vi "Parse Session (Tx-Generic).vi"(8 "error in":errorcluster, 11 "node in":refnum<k20>) -> (0 "error out":errorcluster, 3 "tx_generic_setup":T1={"QueueSizeIn"=0, "Count"=12, "StartMode"=1} {"StartMode" items=["FDX_STOP", "FDX_START", "FDX_START_TRG", "FDX_START_TIME"]})   [LabVIEW 2020, in "AIM ARINC 664 Import.lvlib"]
uses:
  AIM ARINC 664 Import.lvlib
  _typedefs/tx_generic_setup.ctl
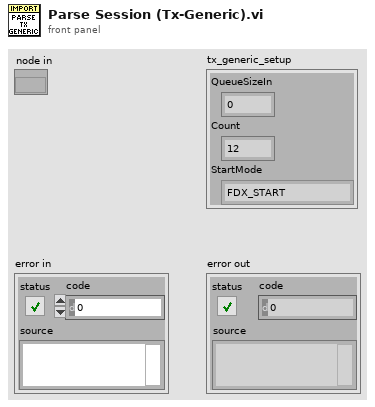
[diagram p1: front panel]
types:
  T1 = typedef "AIM ARINC 664 Import.lvlib/tx_generic_setup.ctl" = cluster{"QueueSizeIn":u32, "Count":i32, "StartMode":i32}
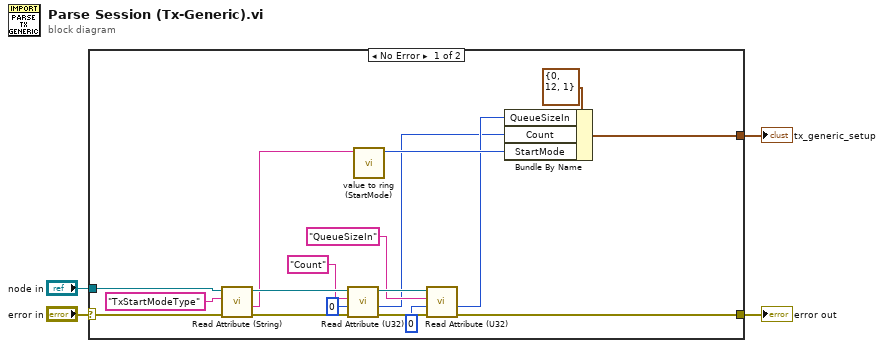
[diagram p0: block diagram]
diagram:
  n1 = case shown="No Error" "error in" {
    selector: "error in" -> [w16 w23]
    tunnel: "node in" -> [w19 _]
    tunnel: [w13 w23] -> w3
    tunnel: [w21 _] -> w1
    frame No Error {
      n2 = call "Read Attribute (String).vi"("error in"=w16, "Attribute Name"="TxStartModeType" ("Name"), "node in"=w19) -> ("error out"=w15:errorcluster, "value"=w7:string, "node out"=w18:refnum<k20>)  [unwired: 6 in]
      n3 = call "Read Attribute (U32).vi"("error in"=w15, "default"=u32 0, "Attribute Name"="Count" ("Tag Name"), "node in"=w18) -> ("error out"=w14:errorcluster, "value"=w8:u32, "node out"=w17:refnum<k20>)  [unwired: 5 in]
      n4 = call "value to ring (StartMode).vi"("value"=w7) -> ("StartMode"=w20:i32)  [unwired: 10 in]
      n5 = call "Read Attribute (U32).vi"("error in"=w14, "default"=u32 0, "Attribute Name"="QueueSizeIn" ("Tag Name"), "node in"=w17) -> ("error out"=w13:errorcluster, "value"=w9:u32)  [unwired: 5 in, 1 out]
      n6 = Bundle By Name(cluster=T1 {"QueueSizeIn"=0, "Count"=12, "StartMode"=1} ("tx_generic_setup"), "QueueSizeIn"=w9, "Count"=w8, "StartMode"=w20) -> (w21:T1)
    }
    frame Error {
    }
  }
  "error out" <- w3
  "tx_generic_setup" <- w1
